vi "Write Data Name.vi"(8 "error in (no error)":errorcluster, 10 "Data Name":string, 11 "dataPayload in":refnum<class "dataPayload.lvclass">) -> (0 "error out":errorcluster, 3 "dataPayload out":refnum<class "dataPayload.lvclass">)   [LabVIEW 2017, in "messagesPayload.lvlib" / "dataPayload.lvclass"]
uses:
  dataPayload.lvclass
  dataPayload.lvclass/dataPayload.ctl
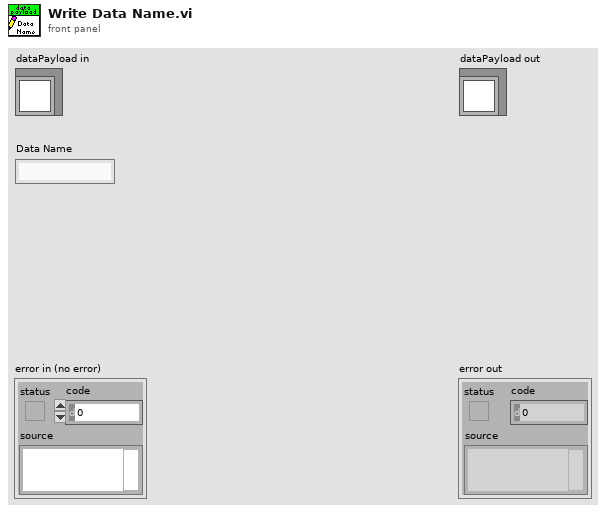
[diagram p1: front panel]
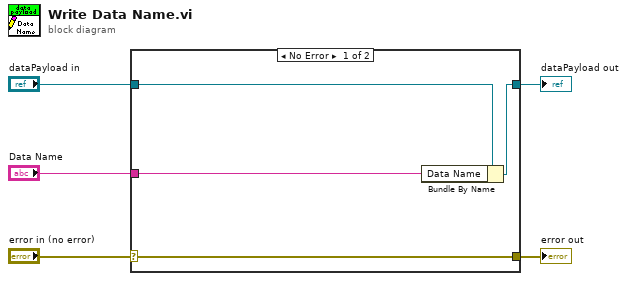
[diagram p0: block diagram]
diagram:
  n1 = case shown="No Error" "error in (no error)" {
    selector: "error in (no error)" -> [w9 w10]
    tunnel: [w9 w10] -> w4
    tunnel: [w7 w11] -> w2
    tunnel: "dataPayload in" -> [w8 w11]
    tunnel: "Data Name" -> [w6 _]
    frame No Error {
      n2 = Bundle By Name(cluster=w8, "Data Name"=w6) -> (w7:refnum<class "dataPayload.lvclass">)
    }
    frame Error {
    }
  }
  "error out" <- w4
  "dataPayload out" <- w2
